vi "_ExtractXMLElementByTag.vi"(4 "error in":errorcluster, 6 "TagName":string, 7 "XML String":string) -> (0 "error out":errorcluster, 1 "TailingString":string, 2 "Element":string, 3 "LeadingString":string)   [LabVIEW 2015]
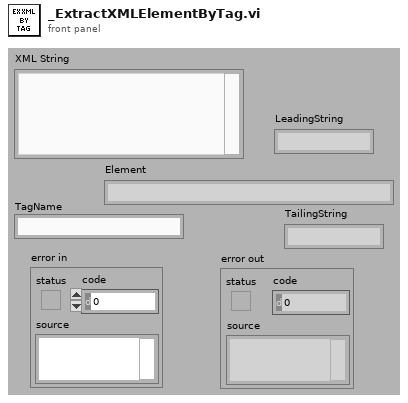
[diagram p1: front panel]
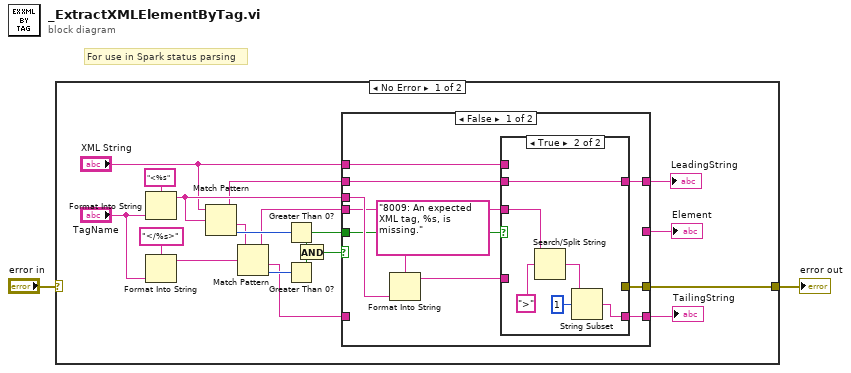
[diagram p0: block diagram]
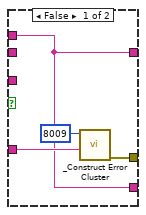
[diagram p2: hidden frame]
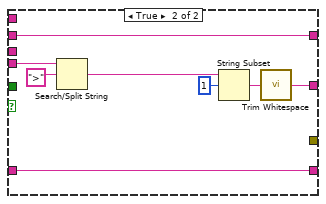
[diagram p3: hidden frame]
diagram:
  # "For use in Spark status parsing"
  n1 = case shown="No Error" "error in" {
    selector: "error in" -> [_ w50]
    tunnel: [w20 w50] -> w1
    frame No Error {
      n2 = Format Into String(format string="<%s", "TagName") -> (resulting string=w13:string)  [unwired: 2 in, 1 out]
      n3 = Format Into String(format string="</%s>", "TagName") -> (resulting string=w11:string)  [unwired: 2 in, 1 out]
      n4 = Match Pattern(string="XML String", regular expression=w13) -> (before substring=w3:string, after substring=w19:string, offset past match=w21:i32)  [unwired: 2 out]
      n5 = Match Pattern(string=w19, regular expression=w11) -> (before substring=w16:string, after substring=w12:string, offset past match=w18:i32)  [unwired: 2 out]
      n6 = Greater Than 0?(x=w21) -> (x > 0?=w4:bool)
      n7 = Greater Than 0?(x=w18) -> (x > 0?=w5:bool)
      n8 = And(x=w4, y=w5) -> (x .and. y?=w17:bool)
      n9 = case shown="False" w17 {
        tunnel: w16 -> [w22 w46]
        tunnel: [w31 _] -> w20
        tunnel: "XML String" -> [w26 _]
        tunnel: w13 -> [w30 _]
        tunnel: w12 -> [_ w49]
        tunnel: [w25 w49] -> w10
        tunnel: [w24 w42] -> w9
        tunnel: [_ w48] -> w8
        tunnel: w4 -> [w27 _]
        tunnel: w3 -> [w23 w42]
        frame False {
          n10 = Format Into String(format string="8009: An expected XML tag, %s, is missing.", w30) -> (resulting string=w28:string)  [unwired: 2 in, 1 out]
          n11 = case shown="True" w27 {
            tunnel: [w35 _] -> w31
            tunnel: w28 -> [w34 _]
            tunnel: w26 -> [w32 _]
            tunnel: [w32 w36] -> w25
            tunnel: [w32 w41] -> w24
            tunnel: w23 -> [_ w41]
            tunnel: w22 -> [_ w39]
            frame False {
              n12 = call "_Construct Error Cluster.vi"("reason"=w34, "errorCode"=8009) -> ("error out"=w35:errorcluster)  [unwired: 2 in, 3 out]
            }
            frame True {
              n13 = Search/Split String(string=w39, search string/char (-)=">") -> (match + rest of string=w37:string)  [unwired: 3 out]
              n14 = String Subset(string=w37, offset (0)=1 ("default value 1")) -> (substring=w36:string)  [unwired: 1 out]
            }
          }
        }
        frame True {
          n15 = Search/Split String(string=w46, search string/char (-)=">") -> (match + rest of string=w43:string)  [unwired: 3 out]
          n16 = String Subset(string=w43, offset (0)=1 ("default value 1")) -> (substring=w44:string)  [unwired: 1 out]
          n17 = call <vilib>:"Trim Whitespace.vi"("string"=w44) -> ("trimmed string"=w48:string)  [unwired: 1 in]
        }
      }
      "TailingString" <- w10
      "LeadingString" <- w9
      "Element" <- w8
    }
    frame Error {
    }
  }
  "error out" <- w1
